vi "Init.vi"(8 "error in":errorcluster, 10 "OD Entry":refnum<class "Object Entry.lvclass">, 11 "PDO Communication Parameter in":refnum<class "PDO Communication Parameter.lvclass">) -> (0 "error out":errorcluster, 3 "PDO Communication Parameter out":refnum<class "PDO Communication Parameter.lvclass">)   [LabVIEW 2020, in "CANopen.lvlib" / "PDO Communication Parameter.lvclass"]
uses:
  PDO Communication Parameter.lvclass
  Object Entry/Object Entry.lvclass
  Object Entry/Object Entry.lvclass/Object Entry.ctl
  Sub Object/Sub Object.lvclass/Sub Object.ctl
  PDO Communication Parameter.lvclass/PDO Communication Parameter.ctl
  Sub Object/Get Default Value.vi
  Sub Object/Default Value is null.vi
  Object Entry/Get Index.vi
  Object Entry/Index is null.vi
  Object Entry/Get Access Type.vi
  Object Entry/Access Type is null.vi
  Object Entry/Get Description.vi
  Object Entry/Description is null.vi
  Sub Object/Get Access Type.vi
  Object Entry/Get Sub Objects Dictionary.vi
  Sub Object/Get Sub Index.vi
  Object Entry/Set Sub Objects Dictionary.vi
  Object Entry/Get Object Type.vi
  Sub Object/Access Type is null.vi
  Object Entry/Get or Create Sub Object.vi
  Object Entry/Set Sub Object.vi
  Sub Objects Dictionary/Get Sub Objects.vi
  CANopen.lvlib
  Sub Object/Sub Object.lvclass
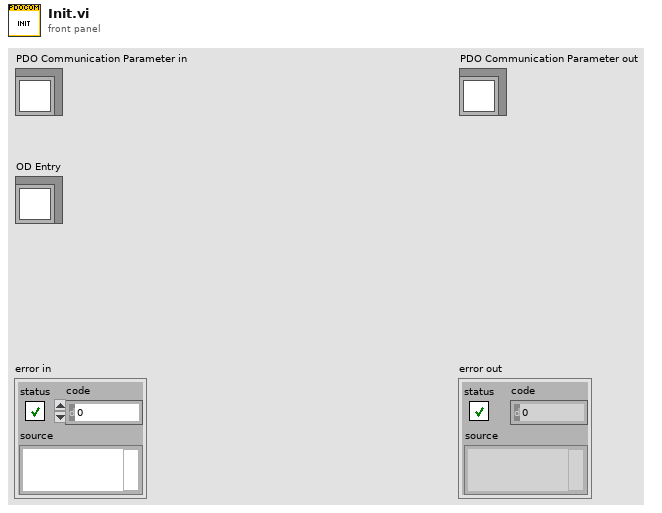
[diagram p1: front panel]
types:
  T1 = typedef "CANopen.lvlib/Access Type.ctl" = enum16{"unknown", "ro", "wo", "rw", "rwr", "rww", "const"}
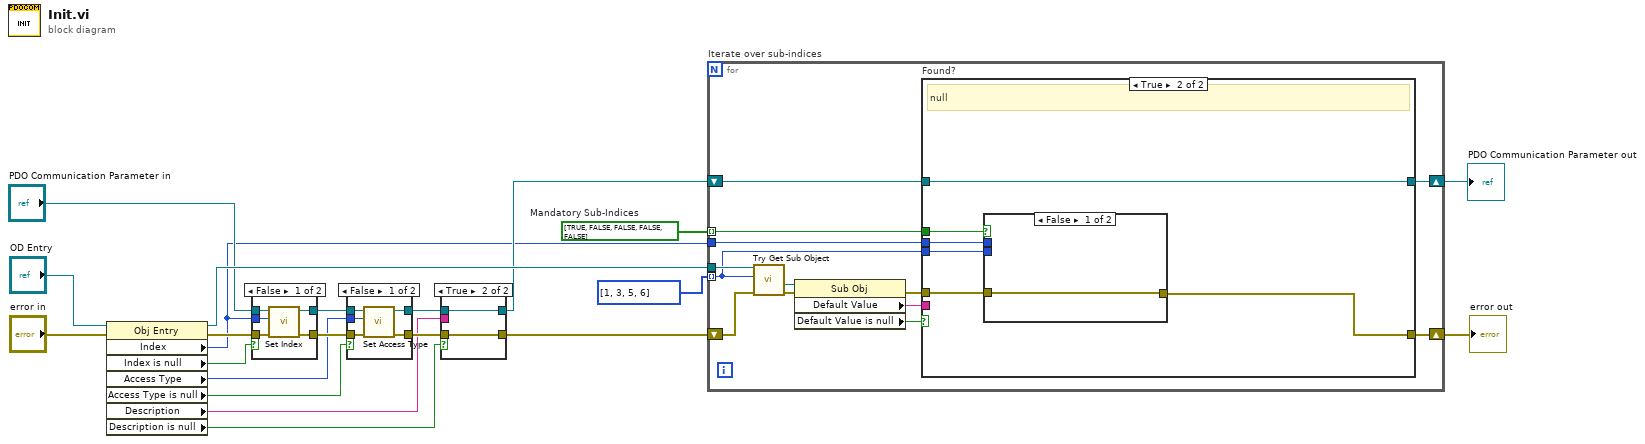
[diagram p0: block diagram]
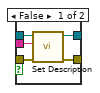
[diagram p2: hidden frame]
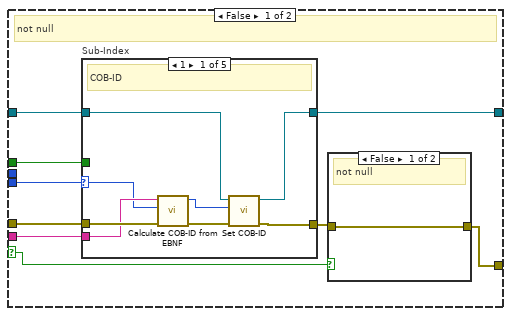
[diagram p5: hidden frame]
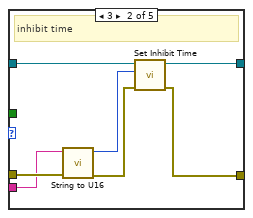
[diagram p6: hidden frame]
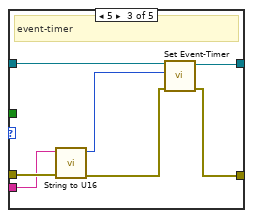
[diagram p7: hidden frame]
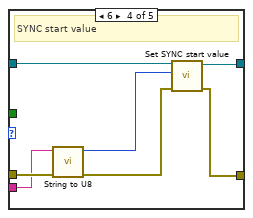
[diagram p8: hidden frame]
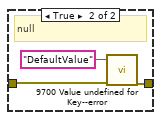
[diagram p10: hidden frame]
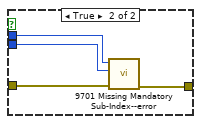
[diagram p11: hidden frame]
diagram:
  w18 = bool[] [TRUE, FALSE, FALSE, FALSE, FALSE]  # Mandatory Sub-Indices
  n1 = property class="Obj Entry"(reference="OD Entry", error in="error in") -> (reference out=w19:refnum<class "Object Entry.lvclass">, error out=w20:errorcluster, "Index"=w1:u16, "Index is null"=w12:bool, "Access Type"=w7:T1, "Access Type is null"=w6:bool, "Description"=w5:string, "Description is null"=w4:bool)
  n2 = case shown="False" w12 {
    tunnel: w20 -> [w26 w27]
    tunnel: [w25 w27] -> w8
    tunnel: "PDO Communication Parameter in" -> [w24 w28]
    tunnel: [w23 w28] -> w11
    tunnel: w1 -> [w22 _]
    frame False {
      n3 = call "Set Index.vi"("error in"=w26, "Index"=w22, "PDO Communication Parameter in"=w24) -> ("error out"=w25:errorcluster, "PDO Communication Parameter out"=w23:refnum<class "PDO Communication Parameter.lvclass">)  [unwired: 7 in]
    }
    frame True {
    }
  }
  n4 = case shown="False" w6 {
    tunnel: w8 -> [w33 w34]
    tunnel: [w32 w34] -> w9
    tunnel: w11 -> [w31 w35]
    tunnel: [w30 w35] -> w10
    tunnel: w7 -> [w29 _]
    frame False {
      n5 = call "Set Access Type.vi"("error in"=w33, "AccessType"=w29, "PDO Communication Parameter in"=w31) -> ("error out"=w32:errorcluster, "PDO Communication Parameter out"=w30:refnum<class "PDO Communication Parameter.lvclass">)  [unwired: 7 in]
    }
    frame True {
    }
  }
  n6 = case shown="True" w4 {
    tunnel: w9 -> [w40 w41]
    tunnel: [w39 w41] -> w3
    tunnel: w10 -> [w38 w42]
    tunnel: [w37 w42] -> w2
    tunnel: w5 -> [w36 _]
    frame False {
      n7 = call "Set Description.vi"("error in"=w40, "Description"=w36, "PDO Communication Parameter in"=w38) -> ("error out"=w39:errorcluster, "PDO Communication Parameter out"=w37:refnum<class "PDO Communication Parameter.lvclass">)  [unwired: 7 in]
    }
    frame True {
    }
  }
  n8 = for "Iterate over sub-indices" {
    tunnel: u8[] [1, 3, 5, 6] -> [w51] mode=indexing
    shift-right: [w54] -> w14
    shift-left: w2 -> [w55]
    shift-right: [w53] -> w15
    shift-left: w3 -> [w50]
    tunnel: w19 -> [w52]
    tunnel: w18 -> [w48] mode=indexing
    tunnel: w1 -> [w43]
    n9 = call "Try Get Sub Object.vi"("error in"=w50, "Sub Index"=w51, "Obj Entry in"=w52) -> ("error out"=w49:errorcluster, "Sub Object"=w46:refnum<class "Sub Object.lvclass">)  [unwired: 5 in, 2 out]
    n10 = property class="Sub Obj"(reference=w46, error in=w49) -> (error out=w47:errorcluster, "Default Value"=w44:string, "Default Value is null"=w45:bool)  [unwired: 1 out]
    n11 = case "Found?" shown="True" w45 {
      selector: w45 -> [w57 _]
      tunnel: w55 -> [w64 w102]
      tunnel: [w63 w102] -> w54
      tunnel: [w60 w103] -> w53
      tunnel: w51 -> [w62 w104]
      tunnel: w47 -> [w58 w105]
      tunnel: w48 -> [w59 w101]
      tunnel: w44 -> [w56 _]
      tunnel: w43 -> [_ w100]
      frame False {
        # "not null"
        n12 = case "Sub-Index" shown="1" w62 {
          selector: w62 -> [w67 _ _ _ _]
          tunnel: w64 -> [w66 w78 w85 w92 w95]
          tunnel: [w71 w77 w84 w91 w95] -> w63
          tunnel: w58 -> [w72 w79 w86 w93 w94]
          tunnel: [w69 w75 w81 w88 w94] -> w61
          tunnel: w59 -> [_ _ _ _ _]
          tunnel: w56 -> [w68 w73 w80 w87 _]
          frame 1 {
            # "COB-ID"
            n13 = call "Calculate COB-ID from EBNF.vi"("error in"=w72, "Node ID"=w67, "ENBF"=w68) -> ("error out"=w70:errorcluster, "COB-ID"=w65:u32)  [unwired: 7 in]
            n14 = call "Set COB-ID.vi"("error in (no error)"=w70, "COB-ID"=w65, "PDO Communication Parameter in"=w66) -> ("error out"=w69:errorcluster, "PDO Communication Parameter out"=w71:refnum<class "PDO Communication Parameter.lvclass">)  [unwired: 7 in]
          }
          frame 3 {
            # "inhibit time"
            n15 = call "String to U16.vi"("error in"=w79, "Integer String"=w73) -> ("error out"=w76:errorcluster, "U16"=w74:u16)  [unwired: 8 in]
            n16 = call "Set Inhibit Time.vi"("error in"=w76, "Inhibit Time"=w74, "PDO Communication Parameter in"=w78) -> ("error out"=w75:errorcluster, "PDO Communication Parameter out"=w77:refnum<class "PDO Communication Parameter.lvclass">)  [unwired: 7 in]
          }
          frame 5 {
            # "event-timer"
            n17 = call "String to U16.vi"("error in"=w86, "Integer String"=w80) -> ("error out"=w82:errorcluster, "U16"=w83:u16)  [unwired: 8 in]
            n18 = call "Set Event-Timer.vi"("error in (no error)"=w82, "Event-Timer"=w83, "PDO Communication Parameter in"=w85) -> ("error out"=w81:errorcluster, "PDO Communication Parameter out"=w84:refnum<class "PDO Communication Parameter.lvclass">)  [unwired: 7 in]
          }
          frame 6 {
            # "SYNC start value"
            n19 = call "String to U8.vi"("error in"=w93, "Integer String"=w87) -> ("error out"=w89:errorcluster, "U8"=w90:u8)  [unwired: 8 in]
            n20 = call "Set SYNC start value.vi"("error in"=w89, "SYNC start value"=w90, "PDO Communication Parameter in"=w92) -> ("error out"=w88:errorcluster, "PDO Communication Parameter out"=w91:refnum<class "PDO Communication Parameter.lvclass">)  [unwired: 7 in]
          }
          frame Default {
            # "can't be reached"
          }
        }
        n21 = case "null?" shown="False" w57 {
          tunnel: w61 -> [w96 w98]
          tunnel: [w96 w99] -> w60
          frame False {
            # "not null"
          }
          frame True {
            # "null"
            n22 = call "9700 Value undefined for Key--error.vi"("error in"=w98, "Argument"="DefaultValue" ("key")) -> ("error out"=w99:errorcluster)  [unwired: 9 in]
          }
        }
      }
      frame True {
        # "null"
        n23 = case shown="False" w101 {
          tunnel: w105 -> [w106 w110]
          tunnel: w104 -> [_ w108]
          tunnel: [w106 w109] -> w103
          tunnel: w100 -> [_ w107]
          frame False {
          }
          frame True {
            n24 = call "9701 Missing Mandatory Sub-Index--error.vi"("error in"=w110, "Sub-Index"=w108, "Index"=w107) -> ("error out"=w109:errorcluster)  [unwired: 8 in]
          }
        }
      }
    }
  }
  "error out" <- w15
  "PDO Communication Parameter out" <- w14
